vi "Run Scoring.vi"(4 "Server":refnum<class "SOL-Server.lvclass">, 5 "Submission DB":refnum<class "Submission DB.lvclass">, 7 "Submission":refnum<class "Submission.lvclass">, 8 "error in (no error)":errorcluster, 9 "Scorer Path":path, 10 "LLB Path":path, 11 "Scorer in":refnum<class "Scorer.lvclass">) -> (0 "error out":errorcluster, 3 "Scorer out":refnum<class "Scorer.lvclass">)   [LabVIEW 2020, in "Summer of LabVIEW.lvlib" / "Scorer.lvclass"]
uses:
  Scorer.lvclass
  Submission/Submission.lvclass
  SOL-Server/SOL-Server.lvclass
  Submission DB/Submission DB.lvclass
  Run Scoring Async.vi
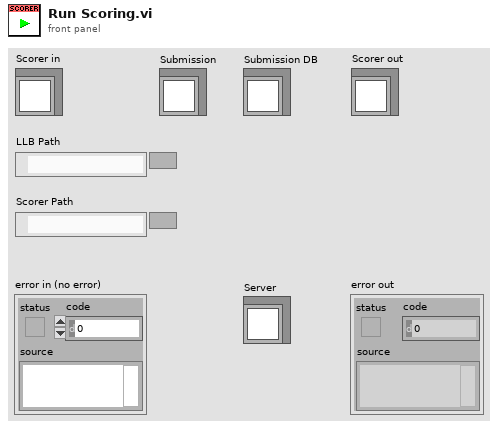
[diagram p1: front panel]
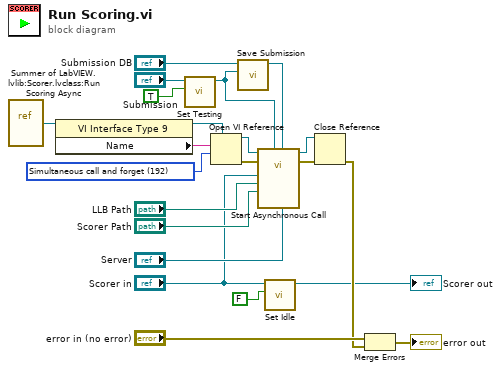
[diagram p0: block diagram]
diagram:
  w16 = 192 items=["Record modifications"=1, "Open templates for editing"=2, "Prompt user to save"=4, "Prepare for reentrant run"=8, "Prompt to find missing subVIs"=16, "Hide loading dialog box"=32, "Enable simultaneous calls"=64, "Prepare to call and forget"=128, "Simultaneous call and forget"=192, "Prepare to call and collect"=256, "Simultaneous call and collect"=320]
  n1 = vi-ref "Summer of LabVIEW.lvlib:Scorer.lvclass:Run Scoring Async.vi"() -> (w14:refnum<vi>)
  n2 = property class="VI Interface Type 9"(reference=w14) -> (reference out=w17:refnum<vi>, "Name"=w15:string)  [unwired: 1 in, 1 out]
  n3 = call "Set Testing.vi"("Testing"=TRUE, "Submission in"="Submission") -> ("Submission out"=w1:refnum<class "Submission.lvclass">)  [unwired: 9 in]
  n4 = Open VI Reference(type specifier VI Refnum (for type only)=w17, vi path=w15, options=w16) -> (vi reference=w19:refnum<vi>, error out=w18:errorcluster)  [unwired: 3 in]
  n5 = call "Save Submission.vi"("Submission"=w1, "Submission DB in"="Submission DB") -> ("Submission DB out"=w2:refnum<class "Submission DB.lvclass">)  [unwired: 8 in, 1 out]
  n6 = call-by-ref "Start Asynchronous Call"(reference=w19, error in=w18, "Server"="Server", "Submission DB"=w2, "Submission"=w1, "Scorer Path"="Scorer Path", "LLB Path"="LLB Path", "Scorer in"="Scorer in") -> (reference out=w21:refnum<vi>, error out=w20:errorcluster)  [unwired: 6 in]
  n7 = call "Set Idle.vi"("Idle"=FALSE, "Scorer in"="Scorer in") -> ("Scorer out"=→"Scorer out":refnum<class "Scorer.lvclass">)  [unwired: 8 in, 1 out]
  n8 = Close Reference(reference=w21, error in (no error)=w20) -> (error out=w10:errorcluster)
  n9 = Merge Errors("error in (no error)", w10) -> (→"error out":errorcluster)
